vi "Generate logfile 3.vi"(9 "Mérés":refnum<vi>, 10 "Teszt vektor listbox":refnum<vi>, 11 "Log_Path":path) -> ()   [LabVIEW 2014]
uses:
  <vilib>/Utility/file.llb/Write To Spreadsheet File (string).vi
panel:
  out "Log line":string[](array[string])
  out "Header":string[](array[string])
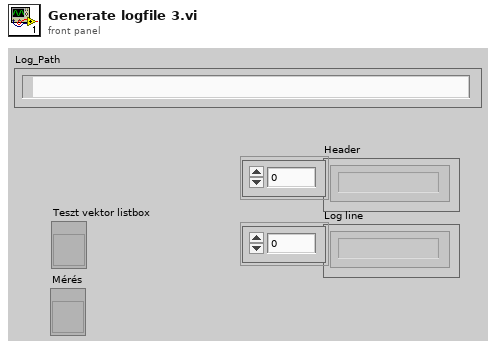
[diagram p1: front panel]
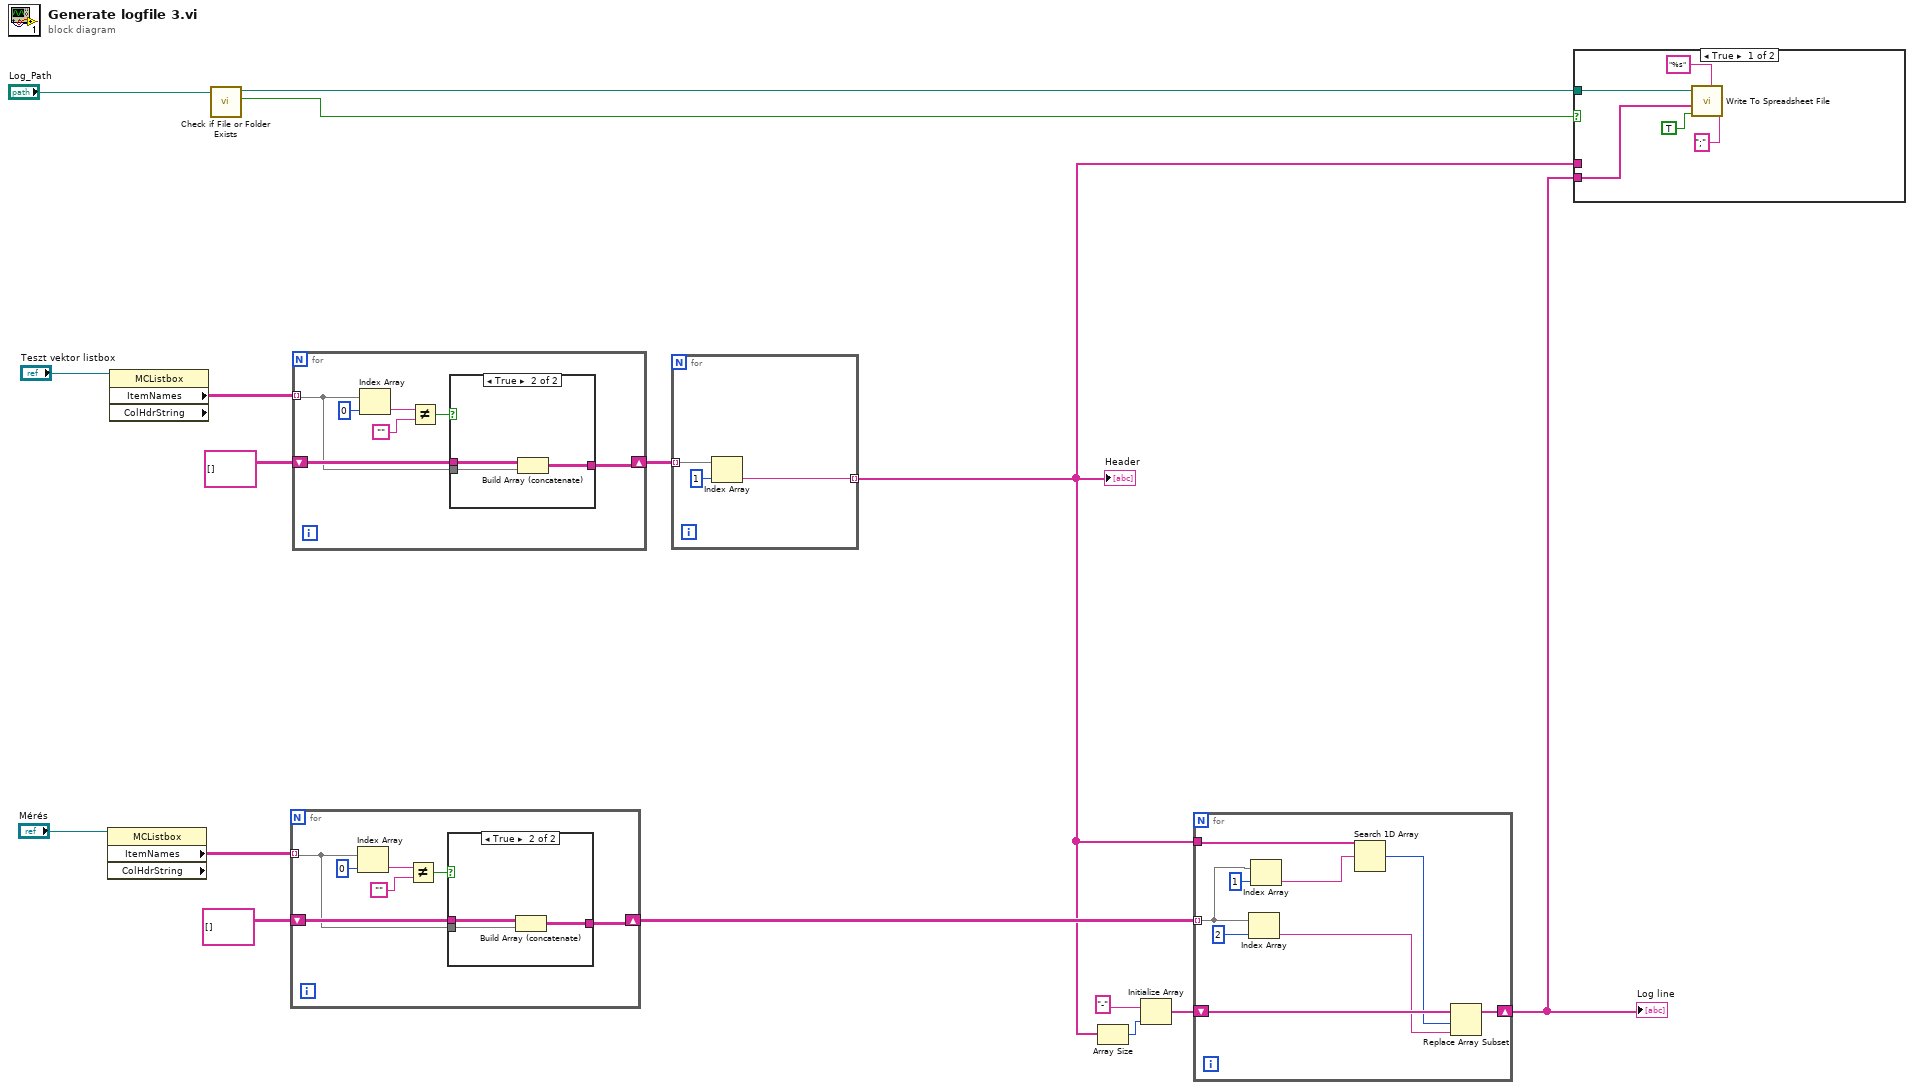
[diagram p0: block diagram]
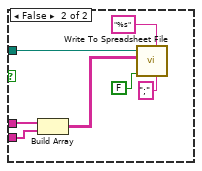
[diagram p2: hidden frame]
diagram:
  n1 = property class="MCListbox" props=["ItemNames", "ColHdrString"](reference="Mérés") -> ("ItemNames"=w11:string[][])  [unwired: 1 in, 3 out]
  n2 = property class="MCListbox" props=["ItemNames", "ColHdrString"](reference="Teszt vektor listbox") -> ("ItemNames"=w15:string[][])  [unwired: 1 in, 3 out]
  n3 = call <vilib>:"Check if File or Folder Exists.vi"("path"="Log_Path") -> ("file or folder exists?"=w8:bool, "dup path"=w7:path)  [unwired: 8 in, 1 out]
  n4 = for {
    tunnel: w11 -> [w18] mode=indexing
    shift-right: [w17] -> w6
    shift-left: string[][] [] ("Item Names") -> [w19]
    n5 = Index Array(array=w18, index=0) -> (element=w22:string)
    n6 = Not Equal?(x=w22, y="") -> (x != y?=w20:bool)
    n7 = case shown="True" w20 {
      tunnel: w19 -> [w24 w27]
      tunnel: w18 -> [_ w26]
      tunnel: [w24 w25] -> w17
      frame False {
      }
      frame True {
        n8 = Build Array (concatenate)(w27, w26) -> (w25:string[][])
      }
    }
  }
  n9 = for {
    tunnel: w15 -> [w29] mode=indexing
    shift-right: [w28] -> w13
    shift-left: string[][] [] ("Item Names") -> [w30]
    n10 = Index Array(array=w29, index=0) -> (element=w33:string)
    n11 = Not Equal?(x=w33, y="") -> (x != y?=w31:bool)
    n12 = case shown="True" w31 {
      tunnel: w30 -> [w35 w38]
      tunnel: w29 -> [_ w37]
      tunnel: [w35 w36] -> w28
      frame False {
      }
      frame True {
        n13 = Build Array (concatenate)(w38, w37) -> (w36:string[][])
      }
    }
  }
  n14 = for {
    tunnel: w13 -> [w41] mode=indexing
    tunnel: [w39] -> w1 mode=indexing
    n15 = Index Array(array=w41, index=1) -> (element=w39:string)
  }
  "Header" <- w1
  n16 = Array Size(array=w1) -> (size(s)=w4:i32)
  n17 = Initialize Array("-", w4) -> (w3:string[])
  n18 = for {
    tunnel: w6 -> [w44] mode=indexing
    shift-right: [w49] -> w2
    shift-left: w3 -> [w50]
    tunnel: w1 -> [w43]
    n19 = Index Array(array=w44, index=2) -> (element=w47:string)
    n20 = Index Array(array=w44, index=1) -> (element=w46:string)
    n21 = Search 1D Array(1D array=w43, element=w46) -> (index of element=w42:i32)  [unwired: 1 in]
    n22 = Replace Array Subset(array=w50, new element=w47, index=w42) -> (w49:string[])
  }
  "Log line" <- w2
  n23 = case shown="True" w8 {
    tunnel: w7 -> [w55 w62]
    tunnel: w1 -> [_ w60]
    tunnel: w2 -> [w52 w59]
    frame True {
      n24 = call-poly <vilib>:"Write To Spreadsheet File.vi"("delimiter (\\t)"=";" ("delimiter (\\t)"), "format (%s)"="%s" ("format (%.3f)"), "append to file? (new file:F)"=TRUE, "1D data"=w52, "file path (dialog if empty)"=w55) -> ()  [unwired: 3 in, 1 out]
    }
    frame False {
      n25 = Build Array(w60, w59) -> (w58:string[][])
      n26 = call-poly <vilib>:"Write To Spreadsheet File.vi"("delimiter (\\t)"=";" ("delimiter (\\t)"), "format (%s)"="%s", "append to file? (new file:F)"=FALSE, "2D data"=w58, "file path (dialog if empty)"=w62) -> ()  [unwired: 3 in, 1 out]
    }
  }
